vi "Teststand Read Variables.vi"(8 "error in":errorcluster, 11 "Sequence Context In":refnum<k7>) -> (0 "error out":errorcluster)   [LabVIEW 2023, in "HardwareAbstractionLayer_LVOOP.lvlib" / "Teststand.lvclass"]
uses:
  Teststand.lvclass
  Control/Teststand Status Control.ctl
  Teststand.lvclass/Teststand.ctl
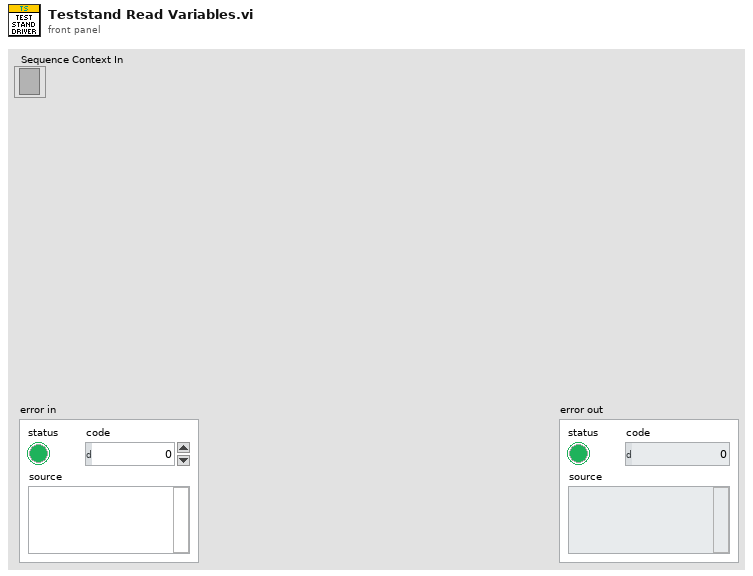
[diagram p1: front panel]
types:
  T1 = typedef "HardwareAbstractionLayer_LVOOP.lvlib/Teststand.lvclass/Teststand Status Control.ctl" = cluster{"Terminating or Aborting":bool, "Stop":bool, "Socket Count":i16, "Selected Sockets":i16[]}
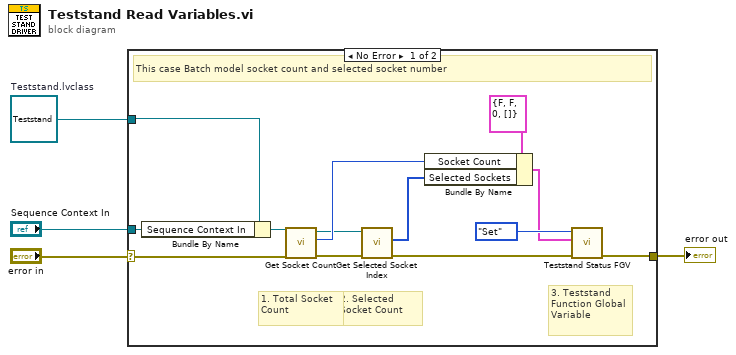
[diagram p0: block diagram]
diagram:
  w2 = refnum<class "Teststand.lvclass"> refnum  # Teststand.lvclass
  n1 = case shown="No Error" "error in" {
    selector: "error in" -> [w14 w18]
    tunnel: [w17 w18] -> w4
    tunnel: "Sequence Context In" -> [w16 _]
    tunnel: w2 -> [w15 _]
    frame No Error {
      # "3. Teststand Function Global Variable"
      # "2. Selected Socket Count"
      # "1. Total Socket Count"
      # "This case Batch model socket count and selected socket number"
      n2 = Bundle By Name(cluster=w15, "Sequence Context In"=w16) -> (w9:refnum<class "Teststand.lvclass">)
      n3 = call-dynamic "Get Socket Count.vi"("error in (no error)"=w14, "Teststand in"=w9) -> ("error out"=w7:errorcluster, "Socket Count"=w10:i16, "Teststand out"=w8:refnum<class "Teststand.lvclass">)  [unwired: 7 in]
      n4 = call-dynamic "Get Selected Socket Index.vi"("error in (no error)"=w7, "Teststand in"=w8) -> ("error out"=w6:errorcluster, "Slected Scokets"=w5:i16[])  [unwired: 7 in, 1 out]
      n5 = Bundle By Name(cluster=T1 {"Terminating or Aborting"=FALSE, "Stop"=FALSE, "Socket Count"=0, "Selected Sockets"=[]} ("Teststand Status"), "Socket Count"=w10, "Selected Sockets"=w5) -> (w11:T1)
      n6 = call "Teststand Status FGV.vi"("error in"=w6, "Teststand Status"=w11, "Option"=enum16{"Set", "Get"}."Set") -> ("error out"=w17:errorcluster)  [unwired: 7 in, 1 out]
    }
    frame Error {
    }
  }
  "error out" <- w4
